vi "Find Choice ID.vi"(8 "error in (no error)":errorcluster, 11 "Enum":string) -> (0 "error out":errorcluster, 3 "Choice ID":string)   [LabVIEW 2013]
doc: "This vi Search for choice id in database choice table and if not available then add Choice in table\nInput:\n1. Enum Items (eg. Test1,Test2,Test3 in this format)\n2. Error in\n\nOutput:\n1. Error out"
panel:
  out "subarray":string[](array[string])
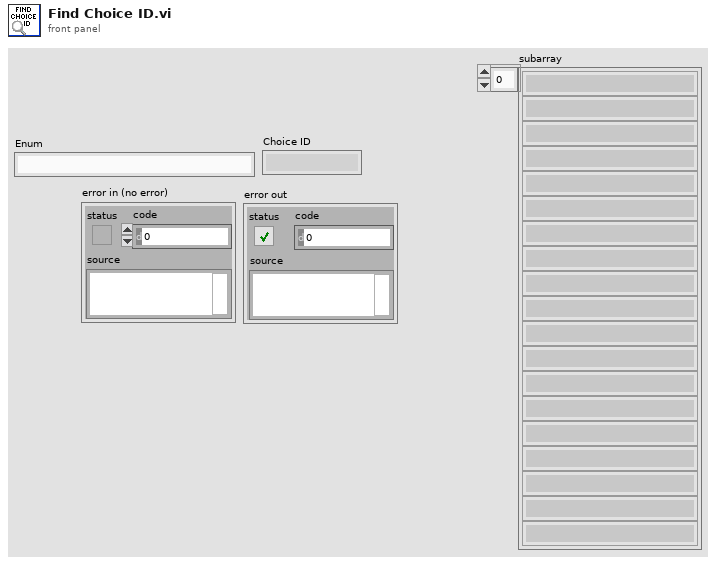
[diagram p1: front panel]
types:
  T1 = typedef "mysql_authentication.ctl" = cluster{"User":string, "Password":string, "Database":string}
  T2 = cluster{"Port":u16, "IP Address":string, "Authentication":T1}
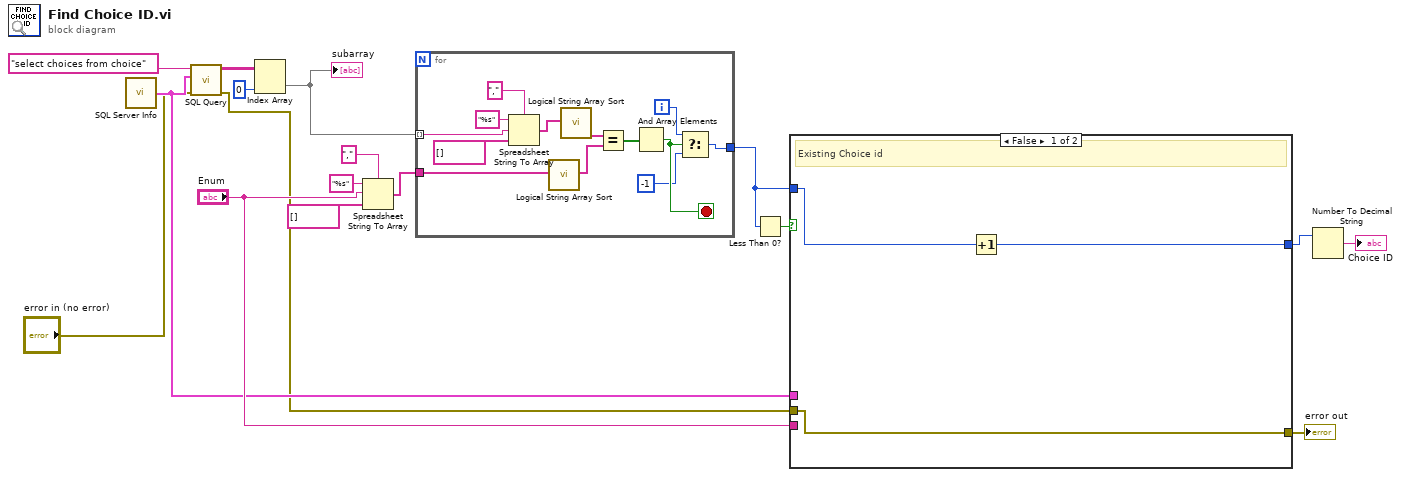
[diagram p0: block diagram]
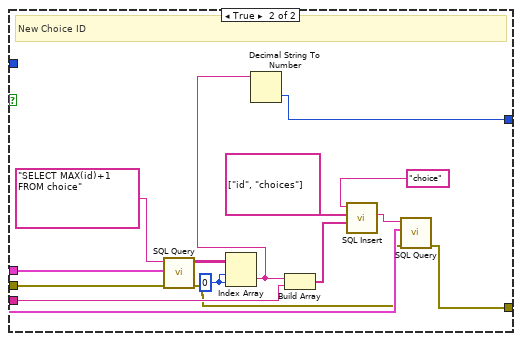
[diagram p2: hidden frame]
diagram:
  n1 = call "SQL Server Info.vi"() -> ("SQL Server Info"=w8:T2)
  n2 = call "SQL Query.vi"("error in (no error)"="error in (no error)", "SQL Server Info"=w8, "Query"="select choices from choice") -> ("error out"=w2:errorcluster, "data"=w15:string[][])  [unwired: 7 in]
  n3 = Index Array(array=w15, index (col)=0 ("disabled index (col)")) -> (element=w10:string[])  [unwired: 1 in]
  "subarray" <- w10
  n4 = Spreadsheet String To Array(delimiter (Tab)=",", format string="%s", spreadsheet string="Enum", array type (2D Dbl)=string[] []) -> (array=w11:string[])
  n5 = for {
    tunnel: w11 -> [w30]
    tunnel: w10 -> [w23] mode=indexing
    tunnel: [w18] -> w6
    i -> [w19]
    stop <- w21 stop-if-true
    n6 = Spreadsheet String To Array(delimiter (Tab)=",", format string="%s", spreadsheet string=w23, array type (2D Dbl)=string[] []) -> (array=w22:string[])
    n7 = call "Logical String Array Sort.vi"("Unsorted List"=w30) -> ("Sorted List"=w29:string[])  [unwired: 18 in]
    n8 = call "Logical String Array Sort.vi"("Unsorted List"=w22) -> ("Sorted List"=w27:string[])  [unwired: 18 in]
    n9 = Equal?(x=w27, y=w29) -> (x = y?=w28:bool[])
    n10 = And Array Elements(Boolean array=w28) -> (logical AND=w21:bool)
    n11 = Select(t=w19, s=w21, f=-1 ("y")) -> (s? t:f=w18:i32)
  }
  n12 = Less Than 0?(x=w6) -> (x < 0?=w7:bool)
  n13 = case shown="False" w7 {
    tunnel: "Enum" -> [_ w41]
    tunnel: w8 -> [_ w39]
    tunnel: w6 -> [w33 _]
    tunnel: [w31 w34] -> w5
    tunnel: w2 -> [w32 w37]
    tunnel: [w32 w36] -> w1
    frame False {
      # "Existing Choice id"
      n14 = Increment(x=w33) -> (x+1=w31:i32)
    }
    frame True {
      w46 = 0 ("disabled index (col)")
      # "New Choice ID"
      n15 = call "SQL Query.vi"("error in (no error)"=w37, "SQL Server Info"=w39, "Query"="SELECT MAX(id)+1 FROM choice") -> ("error out"=w35:errorcluster, "data"=w45:string[][])  [unwired: 7 in]
      n16 = Index Array(array=w45, index (row)=w46, index (col)=w46) -> (element=w38:string)
      n17 = Decimal String To Number(string=w38) -> (number=w34:i32)  [unwired: 2 in, 1 out]
      n18 = Build Array(w38, w41) -> (w40:string[])
      n19 = call "SQL Insert.vi"("Values"=w40, "Column Names"=string[] ["id", "choices"], "Table"="choice") -> ("Query String"=w43:string)  [unwired: 8 in]
      n20 = call "SQL Query.vi"("error in (no error)"=w35, "SQL Server Info"=w39, "Query"=w43) -> ("error out"=w36:errorcluster)  [unwired: 7 in, 1 out]
    }
  }
  "error out" <- w1
  n21 = Number To Decimal String(number=w5) -> (decimal integer string=→"Choice ID":string)  [unwired: 1 in]
